vi "Dashboard Main.vi"() -> ()   [LabVIEW 2013]
uses:
  <vilib>/event_ctls.llb/eventvkey.ctl
  <vilib>/Rock Robotics/WPI/Dashboard/WPI_DashboardLogging Global.vi
  <vilib>/Utility/config.llb/Write Key (String).vi
  <vilib>/Utility/config.llb/Write Key (I32).vi
  <vilib>/Utility/config.llb/NI_LVConfig.lvlib
panel:
  out "Image Message":string="Timeout in Camera Communications"
  in  "Rec Mode":enum32{"Stop", "Record", "Playback"}(radio)
  in  "Dashboard Tab":T1(tab)
  in  "Camera Settings":T2={"Frame Rate"=30, "Compression"=30, "Size"=1} {"Frame Rate" scale=1.0..30.0; "Size" items=["640x480", "320x240", "160x120"]}
  out "MotorSliders R":cluster{"MotorSlide1":dbl, "MotorSlide2":dbl} {"MotorSlide2" scale=-1.0..1.0 scale format="%#_2e"; "MotorSlide1" scale=-1.0..1.0 scale format="%#_2e"}
  out "MotorChart R":cluster{"Numeric":dbl, "Numeric":dbl}(graph)
  out "MotorSliders L":T3 {"MotorSlide4 2" scale=0.0..14.0 scale format="%#_2e"; "MotorSlide2" scale=-1.0..1.0 scale format="%#_2e"; "MotorSlide1" scale=-1.0..1.0 scale format="%#_2e"}
  out "MotorChart L":T4(graph)
  out "JS1 Z":dbl(slide) scale=-1.0..1.0 scale format="%#_2e"
  out "Joystick 1":cluster{"X":dbl, "Y":dbl}[](graph)
  out "JS Buttons 1":T5
  out "JS2 Z":dbl(slide) scale=-1.0..1.0 scale format="%#_2e"
  out "Joystick 2":cluster{"X":dbl, "Y":dbl}[](graph)
  out "JS Buttons 2":T5
  out "Mode":T6(ring)=enum."Auto Disabled"
  out "Camera IP":string
  in  "DB Camera Config":bool
  out "fps":dbl format="%#.1g"
  out "Mbps":dbl format="%#.1g"
  out "Mbps 2":bool
  out "LED 1":bool
  out "Time":string
  in  "Slider 1":dbl(slide) scale=0.0..100.0
  in  "Checkbox 2":bool
  in  "Checkbox 1":bool
  in  "Test Slider":dbl(slide) scale=0.0..100.0 scale format="%#_3g"
  in  "On/Off":bool caption="Solenoid"
  in  "Test Name":u16(ring) items=["Select the test to run...", "Example Test", "-------------------------------", "List of tests is built in robot code.", "Replace with your own automated tests."]
  in  "Test Tree":string(tree)
  in  "Motor":cluster{"Value":dbl, "Enable":bool} {"Value" scale=-1.0..1.0 scale format="%#_3g"}
  out "Progress":T7 {"Test Progress" scale=0.0..100.0}
  in  "Rev/Fwd":cluster{"Forward":bool, "Reverse":bool}
  in  "Test Ring":u16(ring) items=["Auto", "Fixed indoor", "Fixed outdoor 1", "Fixed outdoor 2", "Fixed fluorescent 1", "Fixed fluorescent 2", "Hold current"]
  in  "Listbox":i32(listbox)
  out "Tree":string(tree)
  out "Camera Image":T8(plugin-control)
  in  "Enable":bool
  # "Left"
  # "Front"
  # "Right"
  # "Battery"
  # "Customize by placing controls and indicators here and name to\nmatch Dashboard Variables on robot."
  # "This tab is a great place for autonomous settings and validation.\nCustomize by placing controls and indicators here and name to\nmatch Dashboard Variables on robot."
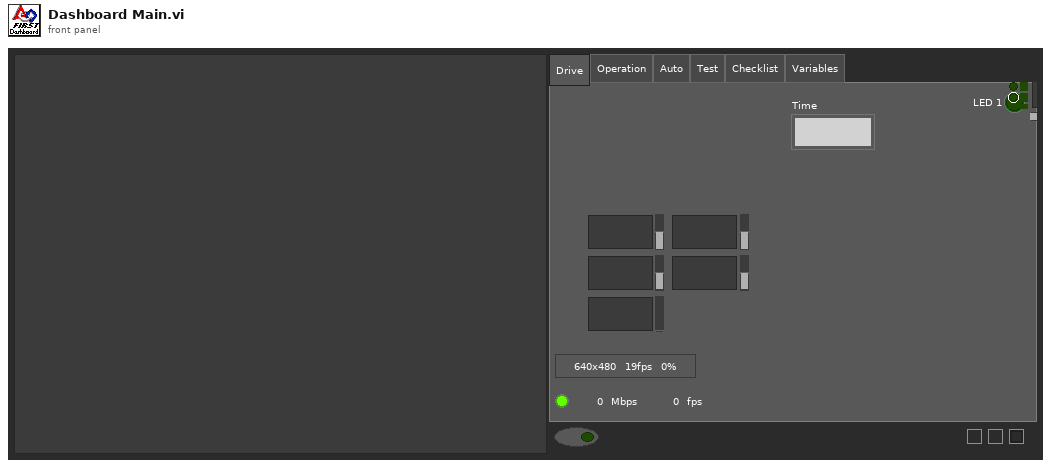
[diagram p1: front panel]
types:
  T1 = enum32{"Drive", "Operation", "Auto", "Test", "Checklist", "Variables"}
  T2 = cluster{"Frame Rate":i32, "Compression":i32, "Size":u16}
  T3 = cluster{"MotorSlide1":dbl, "MotorSlide2":dbl, "MotorSlide4 2":dbl}
  T4 = cluster{"Numeric":dbl, "Numeric":dbl, "Battery":sgl}
  T5 = cluster{bool, bool, bool, bool, bool, bool, bool, bool, bool, bool, bool, bool}
  T6 = enum8{"Tele-Op Disabled", "Tele-Op Enabled", "Auto Disabled", "Auto Enabled", "Test Disabled", "Test Enabled", ""}
  T7 = cluster{"Test Progress":u8, "Test Progress Text":string}
  T8 = typedef "IMAQ Image.ctl" = refnum<image>
  T9 = typedef "Image Type" = u32
  T10 = cluster{"Digital Inputs":bool[], "Digital Outputs":bool[]}
  T11 = cluster{"Competition mode":bool, "Robot Link":bool, "Autonomous":bool, "Enabled":bool, "E-Stop":bool, "Simulated":bool, "TestMode":bool, "Docked Window":bool}
  T12 = cluster{"Boolean Array[0]":bool, "Boolean Array[1]":bool, "Boolean Array[2]":bool, "Boolean Array[3]":bool, "Boolean Array[4]":bool, "Boolean Array[5]":bool, "Boolean Array[6]":bool, "Boolean Array[7]":bool, "Boolean Array[8]":bool, "Boolean Array[9]":bool, "Boolean Array[10]":bool, "Boolean Array[11]":bool}
  T13 = typedef "NI_LVConfig.lvlib/Config Data RefNum.ctl" = refnum<k1>
  T14 = typedef "eventvkey.ctl" = enum16{"ASCII", "Enter", "Return", "Shift", "Ctrl", "Alt", "Cmd", "Opt", "Caps", "NumLock", "Clear", "Break", "Up", "Down", "Left", "Right", "Insert", "Delete", "Home", "End", "PageUp", "PageDown", "Escape", "Help", "Pause", "ScrollLock", "F1", "F2", "F3", "F4", "F5", "F6", "F7", "F8", "F9", "F10", "F11", "F12", "F13", "F14", "F15", "F16", "F17", "F18", "F19", "F20", "F21", "F22", "F23", "F24", "Play", "VolumeUp", "VolumeDown", "Mute", "Two Byte Char"}
  T15 = cluster{"Image Size":bool, "Image Type":bool, "Pixel Value":bool, "ROI Information":bool, "Zoom Factor":bool}
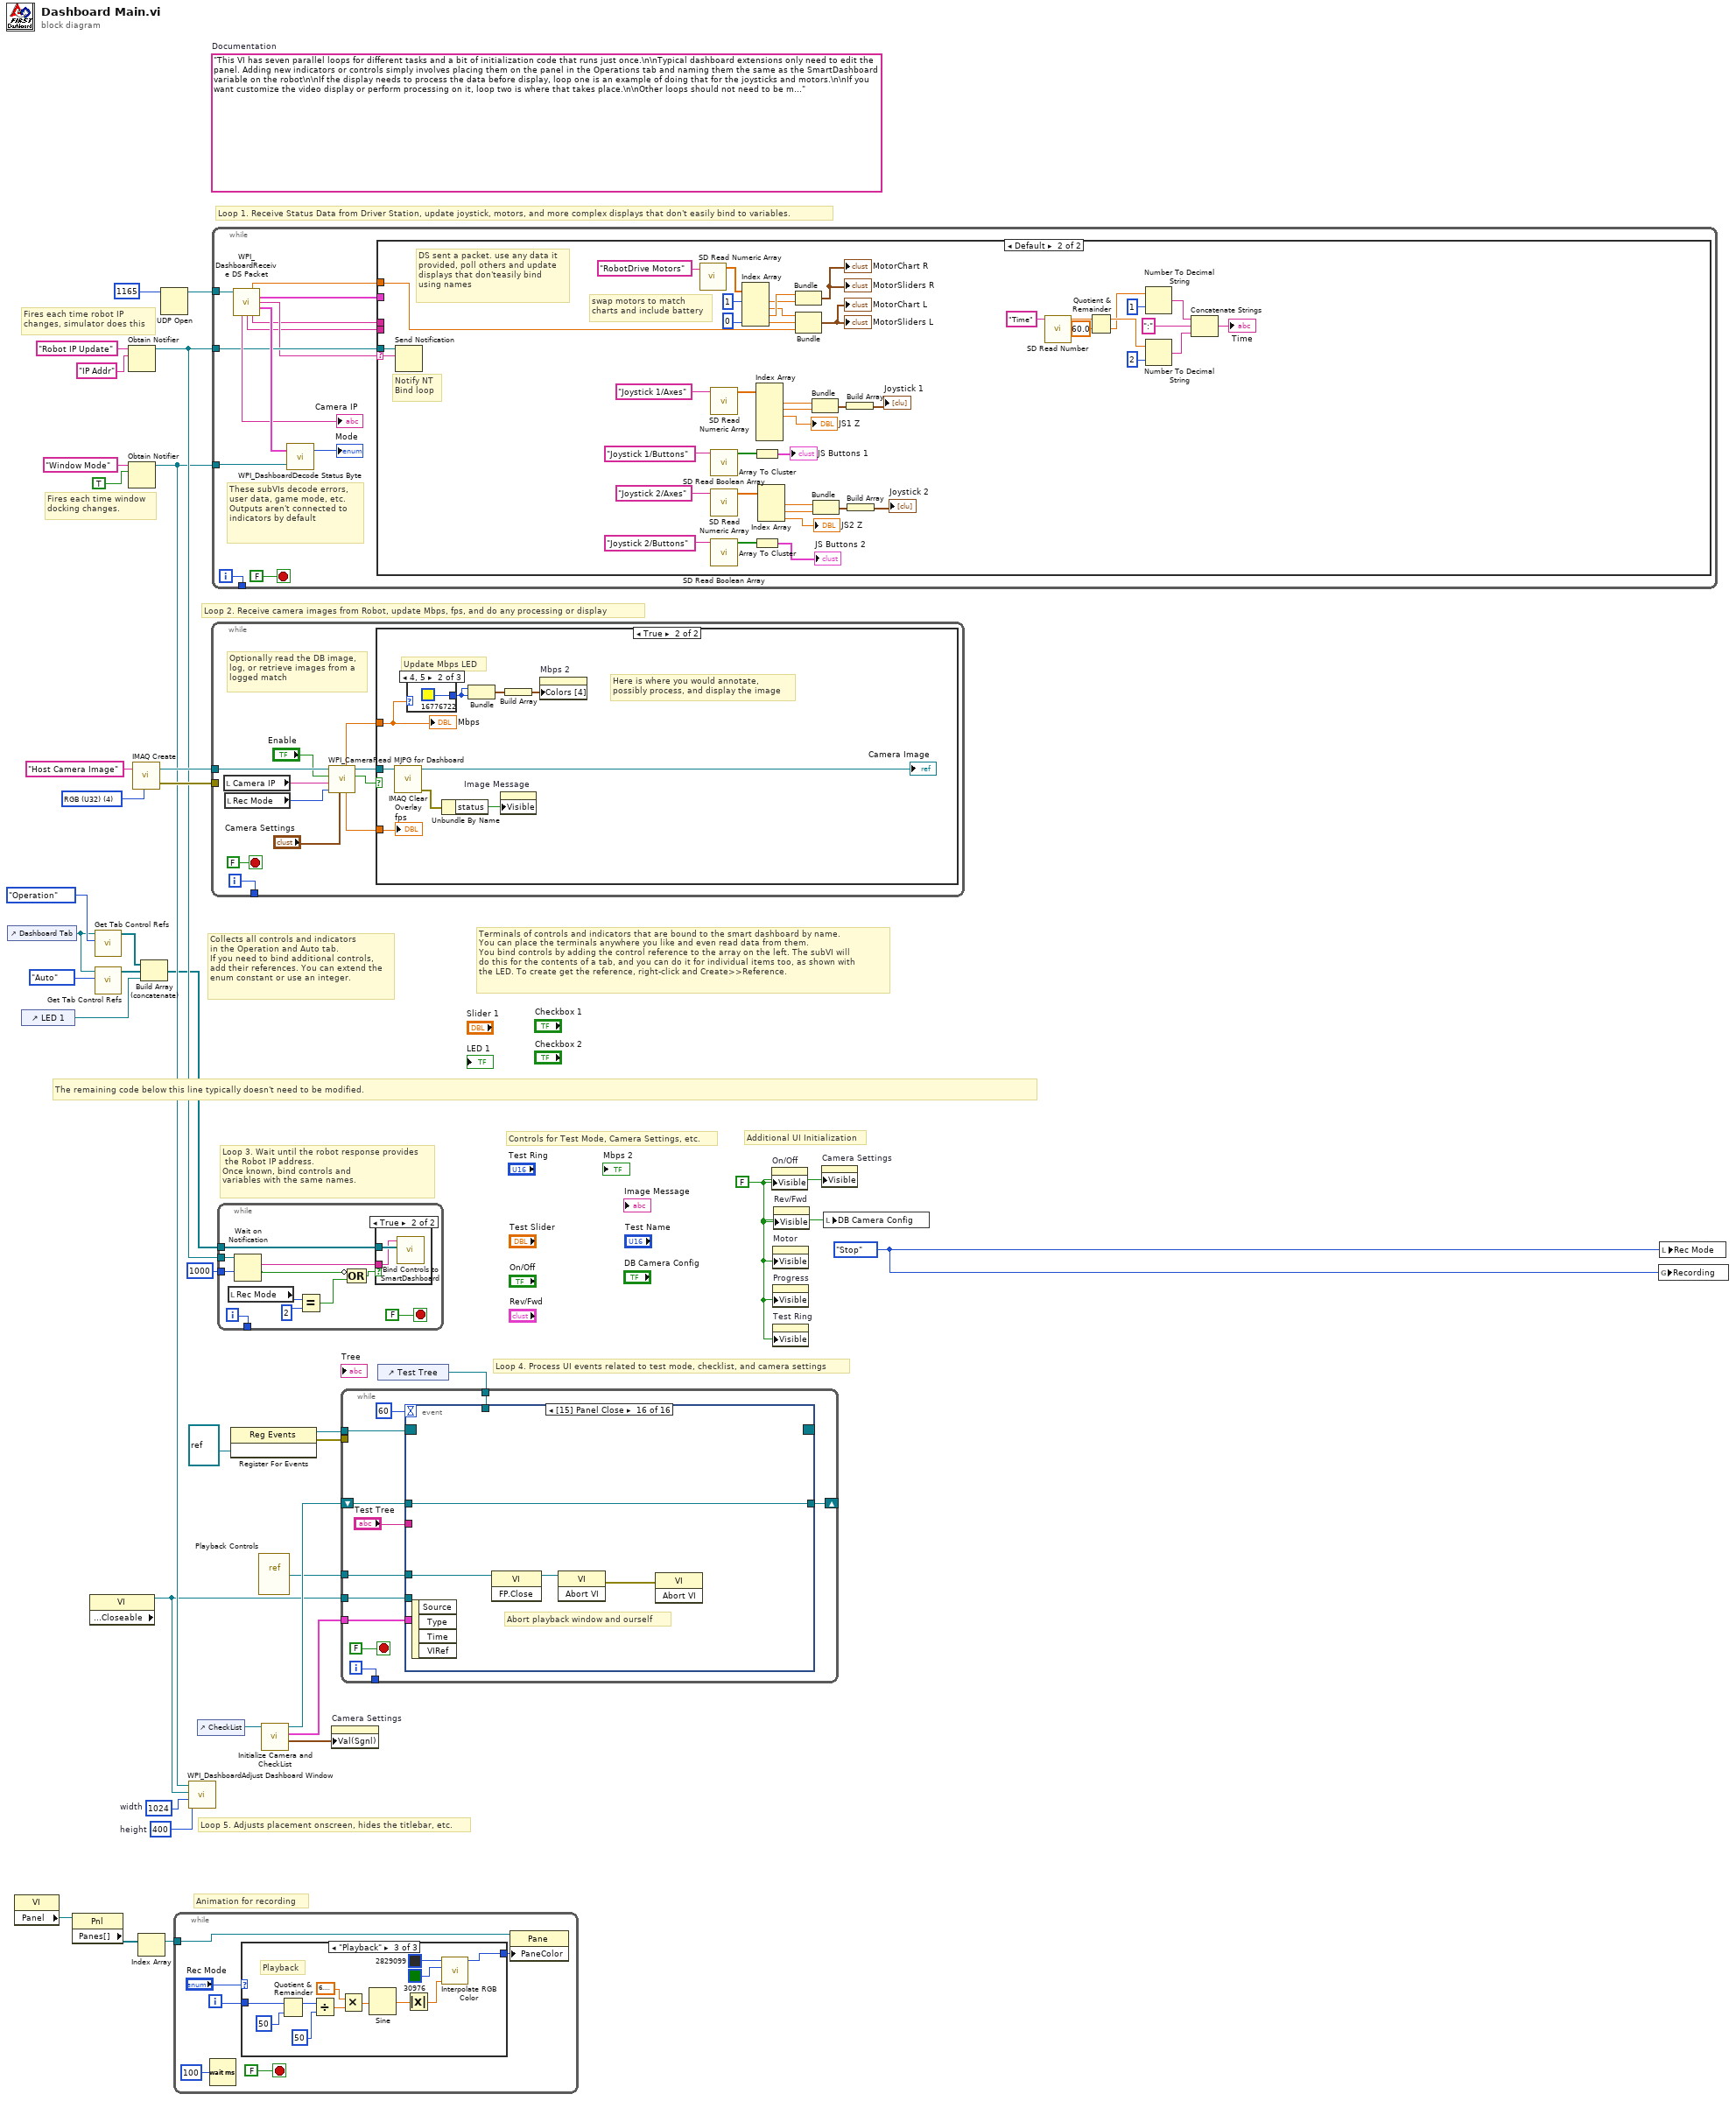
[diagram p0: block diagram]
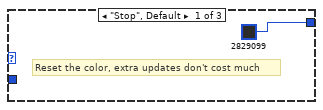
[diagram p2: hidden frame]
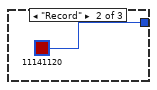
[diagram p3: hidden frame]
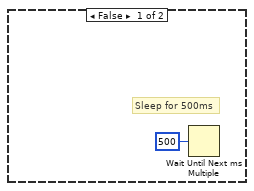
[diagram p5: hidden frame]
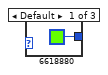
[diagram p6: hidden frame]
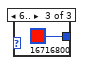
[diagram p7: hidden frame]
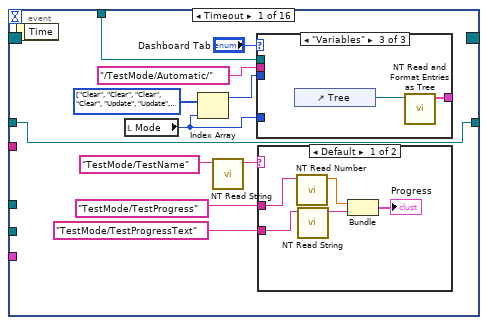
[diagram p8: hidden frame]
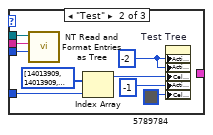
[diagram p10: hidden frame]
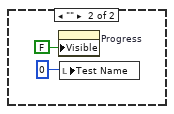
[diagram p11: hidden frame]
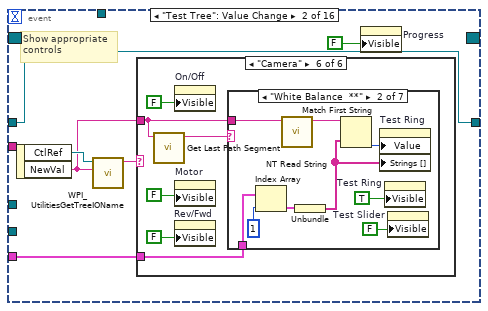
[diagram p12: hidden frame]
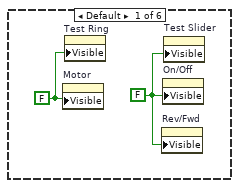
[diagram p13: hidden frame]
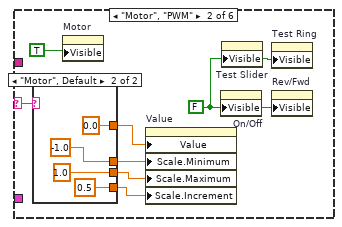
[diagram p14: hidden frame]
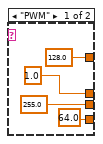
[diagram p15: hidden frame]
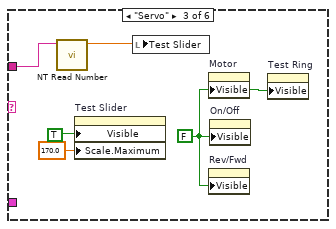
[diagram p16: hidden frame]
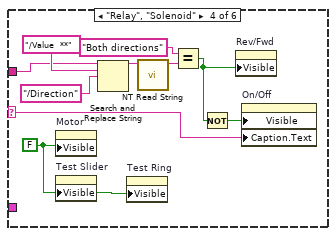
[diagram p17: hidden frame]
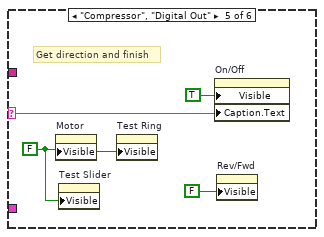
[diagram p18: hidden frame]
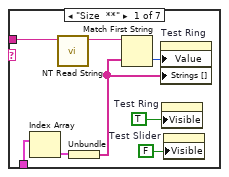
[diagram p19: hidden frame]
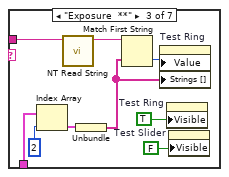
[diagram p20: hidden frame]
diagram:
  w8 = enum32{"Stop", "Record", "Playback"}."Stop" ("Rec Mode")
  w11 = 400  # height
  w12 = 1024  # width
  w25 = FALSE ("Visible")
  (unwired) "This VI has seven parallel loops for different tasks and a bit of initialization code that runs just once.\n\nTypical dashboard extensions only need to edit the panel. Adding new indicators or controls simply involves placing them on the panel in the Operations tab and naming them the same as the SmartDashboard variable on the robot\n\nIf the display needs to process the data before display, loop one is an example of doing that for the joysticks and motors.\n\nIf you want customize the video display or perform processing on it, loop two is where that takes place.\n\nOther loops should not need to be modified. They are pretty standard, and document the task they perform."  # Documentation
  w35 = T9 4 items=["Grayscale (U8)", "Grayscale (I16)", "Grayscale (SGL)", "Complex (CSG)", "RGB (U32)", "HSL (U32)", "RGB (U64)"] ("Image Type")
  # "Controls for Test Mode, Camera Settings, etc."
  # "Additional UI Initialization"
  # "Animation for recording"
  # "Fires each time robot IP\nchanges, simulator does this"
  # "Fires each time window\ndocking changes."
  # "Collects all controls and indicators\nin the Operation and Auto tab.\nIf you need to bind additional controls,\nadd their references. You can extend the\nenum constant or use an integer."
  # "The remaining code below this line typically doesn't need to be modified."
  # "Loop 4. Process UI events related to test mode, checklist, and camera settings"
  # "Terminals of controls and indicators that are bound to the smart dashboard by name.\nYou can place the terminals anywhere you like and even read data from them.\nYou bind controls by adding the control reference to the array on the left. The subVI will\ndo this for the contents of a tab, and you can do it for individual items too, as shown with\nthe LED. To create get the reference, right-click and Create>>Reference."
  # "Loop 3. Wait until the robot response provides\n the Robot IP address.\nOnce known, bind controls and\nvariables with the same names."
  # "Loop 5. Adjusts placement onscreen, hides the titlebar, etc."
  # "Loop 1. Receive Status Data from Driver Station, update joystick, motors, and more complex displays that don't easily bind to variables."
  # "Loop 2. Receive camera images from Robot, update Mbps, fps, and do any processing or display"
  n1 = control-ref of="Dashboard Tab"() -> (w6:refnum<vi>)
  n2 = property class="VI"() -> ("Panel"=w19:refnum<vi>)  [unwired: 2 in, 2 out]
  n3 = control-ref of="LED 1"() -> (w1:refnum<vi>)
  n4 = property class="Pnl"(reference=w19) -> ("Panes[]"=w20:refnum<vi>[])  [unwired: 1 in, 2 out]
  n5 = property class="VI" props=["Front Panel.Closeable"]() -> (reference out=w7:refnum<vi>)  [unwired: 2 in, 2 out]
  n6 = call <vilib>:"Get Tab Control Refs.vi"("Page Index"=T1."Operation" ("Dashboard Tab"), "TabControl in"=w6) -> ("ControlsOnPage"=w4:refnum<vi>[])  [unwired: 9 in]
  n7 = call <vilib>:"Get Tab Control Refs.vi"("Page Index"=T1."Auto" ("Dashboard Tab"), "TabControl in"=w6) -> ("ControlsOnPage"=w5:refnum<vi>[])  [unwired: 9 in]
  n8 = Obtain Notifier(name (unnamed)="Robot IP Update", notification data type="IP Addr" ("name (unnamed)")) -> (notifier out=w29:refnum<notifier>)  [unwired: 2 in, 2 out]
  n9 = Obtain Notifier(name (unnamed)="Window Mode", notification data type=TRUE) -> (notifier out=w10:refnum<notifier>)  [unwired: 2 in, 2 out]
  n10 = call "IMAQ Create"("Image Name"="Host Camera Image", "Image Type"=w35) -> ("New Image"=w33:T8, "error out"=w32:errorcluster)  [unwired: 2 in, 1 out]
  n11 = Index Array(array=w20) -> (element=w18:refnum<vi>)  [unwired: 1 in]
  n12 = Build Array (concatenate)(w4, w5, w1) -> (w3:refnum<vi>[])
  n13 = UDP Open(11:u16 1165 ("port")) -> (port=w36:refnum<k16>)  [unwired: 2 in, 4 out]
  n14 = while {
    tunnel: w18 -> [w39]
    i -> [w42]
    stop <- FALSE stop-if-true
    n15 = Wait (ms)(milliseconds to wait=u32 100) -> ()  [unwired: 1 out]
    n16 = case shown="\"Playback\"" "Rec Mode" {
      tunnel: w42 -> [_ _ w57]
      tunnel: [u32 2829099 ("Base Color") u32 11141120 ("Target Color") w46] -> w38
      frame "Stop", Default {
        # "Reset the color, extra updates don't cost much"
      }
      frame "Record" {
      }
      frame "Playback" {
        # "Playback"
        n17 = Quotient & Remainder(x=w57, y=u32 50 ("milliseconds to wait")) -> (x-y*floor(x/y)=w53:u32)  [unwired: 1 out]
        n18 = Divide(x=w53, y=u32 50 ("milliseconds to wait")) -> (x/y=w50:dbl)
        n19 = Multiply(x=6.283185307179586, y=w50) -> (x*y=w55:dbl)
        n20 = Sine(x=w55) -> (sin(x)=w54:dbl)
        n21 = Absolute Value(x=w54) -> (abs(x)=w47:dbl)
        n22 = call "Interpolate RGB Color.vi"("Proportion"=w47, "Target Color"=u32 30976, "Base Color"=u32 2829099) -> ("Result Color"=w46:u32)  [unwired: 8 in]
      }
    }
    n23 = property class="Pane"(reference=w39, "PaneColor"=w38) -> ()  [unwired: 1 in, 2 out]
  }
  n24 = call <vilib>:"WPI_DashboardAdjust Dashboard Window.vi"("height"=w11, "width"=w12, "reference in"=w7, "Notifier in"=w10) -> ()  [unwired: 8 in]
  n25 = control-ref of="CheckList"() -> (w9:refnum<vi>)
  n26 = while {
    tunnel: w33 -> [w66]
    tunnel: w32 -> [_]
    tunnel: [w67] -> _
    i -> [w67]
    stop <- FALSE stop-if-true
    # "Optionally read the DB image,\nlog, or retrieve images from a\nlogged match"
    n27 = local read "Camera IP"() -> (w59:string)
    n28 = local read "Rec Mode"() -> (w58:enum32{"Stop", "Record", "Playback"})
    n29 = call <vilib>:"WPI_CameraRead MJPG for Dashboard.vi"("Camera Settings"="Camera Settings", "Rec Mode"=w58, "Camera IP"=w59, "Enable"="Enable", "Refnum in"=w66) -> ("Active"=w63:bool, "Refnum out"=w65:T8, "FPS"=w62:dbl, "Bandwidth (Mbps)"=w61:dbl)  [unwired: 3 in]
    n30 = case shown="True" w63 {
      tunnel: w65 -> [_ w73]
      tunnel: w61 -> [_ w72]
      tunnel: w62 -> [_ w70]
      frame False {
        # "Sleep for 500ms"
        n31 = Wait Until Next ms Multiple(millisecond multiple=u32 500) -> ()  [unwired: 1 out]
      }
      frame True {
        # "Here is where you would annotate,\npossibly process, and display the image"
        # "Update Mbps LED"
        n32 = call "IMAQ Clear Overlay"("Image"=w73) -> ("error out"=w77:errorcluster, "Image Out"=→"Camera Image":T8)  [unwired: 2 in, 7 out]
        n33 = case shown="4, 5" w72 {
          tunnel: [u32 6618880 ("Color Box") u32 16776722 ("Color Box") u32 16716800 ("Color Box")] -> w74
          frame Default {
          }
          frame 4, 5 {
          }
          frame 6.. {
          }
        }
        n34 = Unbundle By Name(w77) -> ("status"=w78:bool)
        n35 = Bundle("Color Box"=w74, "Color Box"=w74) -> (w76:cluster{"Color Box":u32, "Color Box":u32})  [unwired: 1 out]
        n36 = property on="Image Message" class="Str"("Visible"=w78) -> ()  [unwired: 2 in, 2 out]
        n37 = Build Array(w76) -> (w75:cluster{"Color Box":u32, "Color Box":u32}[])
        n38 = property on="Mbps 2" class="Bool (strict)"("Colors [4]"=w75) -> ()  [unwired: 2 in, 2 out]
        "Mbps" <- w72
        "fps" <- w70
      }
    }
  }
  n39 = while {
    tunnel: w36 -> [w92]
    tunnel: w29 -> [w87]
    tunnel: w10 -> [w91]
    tunnel: [w88] -> _
    i -> [w88]
    stop <- FALSE stop-if-true
    # "These subVIs decode errors, user data, game mode, etc.\nOutputs aren't connected to indicators by default"
    n40 = call <vilib>:"WPI_DashboardReceive DS Packet.vi"("Recv Socket"=w92) -> ("Battery"=w82:sgl, "Driver Station"=w83:T10, "Robot IP Address"=w86:string, "Status"=w93:T11, "Camera IP Address"=→"Camera IP":string, "Low Priority User Data"=w85:string, "High Priority User Data"=w84:string)  [unwired: 1 in, 7 out]
    n41 = call <vilib>:"WPI_DashboardDecode Status Byte.vi"("Window Mode Notifier"=w91, "Status"=w93) -> ("Mode"=→"Mode":T6)  [unwired: 1 out]
    n42 = case shown="Default" w86 {
      selector: w86 -> [_ w116]
      tunnel: w87 -> [_ w117]
      tunnel: w85 -> [_ _]
      tunnel: w84 -> [_ _]
      tunnel: w83 -> [_ _]
      tunnel: w82 -> [_ w115]
      frame "0.0.0.0" {
        # "DS not sending packets, or no robot exists yet.\nDon't poll the variables"
      }
      frame Default {
        # "Notify NT\nBind loop"
        # "DS sent a packet. use any data it\nprovided, poll others and update\ndisplays that don'teasily bind\nusing names"
        # "swap motors to match\ncharts and include battery"
        n43 = Send Notification(notification=w116, notifier=w117) -> ()  [unwired: 1 in, 2 out]
        n44 = call <vilib>:"SD Read Numeric Array.vi"("Name"="RobotDrive Motors") -> ("Numeric Array"=w114:dbl[])  [unwired: 8 in, 2 out]
        n45 = call <vilib>:"SD Read Numeric Array.vi"("Name"="Joystick 1/Axes") -> ("Numeric Array"=w133:dbl[])  [unwired: 8 in, 2 out]
        n46 = call <vilib>:"SD Read Boolean Array.vi"("Name"="Joystick 1/Buttons") -> ("Boolean Array"=w135:bool[])  [unwired: 8 in, 2 out]
        n47 = call <vilib>:"SD Read Numeric Array.vi"("Name"="Joystick 2/Axes") -> ("Numeric Array"=w127:dbl[])  [unwired: 8 in, 2 out]
        n48 = call <vilib>:"SD Read Boolean Array.vi"("Name"="Joystick 2/Buttons") -> ("Boolean Array"=w126:bool[])  [unwired: 8 in, 2 out]
        n49 = Index Array(array=w114, index #1=1, index #4=0) -> (element #1=w110:dbl, element #2=w109:dbl, element #3=w111:dbl, element #4=w106:dbl)  [unwired: 2 in]
        n50 = Array To Cluster(array=w135) -> (cluster=→"JS Buttons 1":T12)
        n51 = Array To Cluster(array=w126) -> (cluster=→"JS Buttons 2":T12)
        n52 = Index Array(array=w133) -> (element #1=w130:dbl, element #2=w131:dbl, element #3=→"JS1 Z":dbl)  [unwired: 6 in, 3 out]
        n53 = Index Array(array=w127) -> (element #1=w122:dbl, element #2=w121:dbl, element #3=→"JS2 Z":dbl)  [unwired: 3 in]
        n54 = Bundle("Numeric"=w111, "Numeric"=w110) -> (→"MotorChart R" →"MotorSliders R":cluster{"Numeric":dbl, "Numeric":dbl})  [unwired: 1 in]
        n55 = Bundle("Numeric"=w109, "Numeric"=w106, "Battery"=w115) -> (→"MotorChart L" →"MotorSliders L":T4)  [unwired: 1 in]
        n56 = Bundle("Numeric"=w130, "Numeric"=w131) -> (w129:cluster{"Numeric":dbl, "Numeric":dbl})  [unwired: 1 in]
        n57 = Bundle("Numeric"=w122, "Numeric"=w121) -> (w123:cluster{"Numeric":dbl, "Numeric":dbl})  [unwired: 1 in]
        n58 = Build Array(w129) -> (→"Joystick 1":cluster{"Numeric":dbl, "Numeric":dbl}[])
        n59 = Build Array(w123) -> (→"Joystick 2":cluster{"Numeric":dbl, "Numeric":dbl}[])
        n60 = call <vilib>:"SD Read Number.vi"("Name"="Time") -> ("Numeric"=w104:dbl)  [unwired: 8 in, 2 out]
        n61 = Quotient & Remainder(x=w104, y=60.0) -> (x-y*floor(x/y)=w99:dbl, floor(x/y)=w96:dbl)
        n62 = Number To Decimal String(number=w96, width (-)=i16 1) -> (decimal integer string=w102:string)
        n63 = Number To Decimal String(number=w99, width (-)=i16 2) -> (decimal integer string=w101:string)
        n64 = Concatenate Strings(w102, ":", w101) -> (→"Time":string)
      }
    }
  }
  n65 = while {
    tunnel: w3 -> [w149]
    tunnel: w29 -> [w147]
    tunnel: [w145] -> _
    tunnel: u32 1000 ("milliseconds to wait") -> [w144]
    i -> [w145]
    stop <- FALSE stop-if-true
    n66 = local read "Rec Mode"() -> (w140:enum32{"Stop", "Record", "Playback"})
    n67 = Wait on Notification(notifier=w147, timeout in ms (-1)=w144) -> (notification=w146:string, timed out?=w142:bool)  [unwired: 2 in, 2 out]
    n68 = Equal?(x=w140, y=u16 2 ("Rec Mode")) -> (x = y?=w141:bool)
    n69 = Compound Arithmetic op=OR(invert w142, w141) -> (w143:bool)
    n70 = case shown="True" w143 {
      tunnel: w149 -> [_ w151]
      tunnel: w146 -> [_ w150]
      frame False {
      }
      frame True {
        n71 = call <vilib>:"Bind Controls to SmartDashboard.vi"("Bound Control Refs"=w151, "Server IP Address"=w150) -> ()  [unwired: 10 in]
      }
    }
  }
  n72 = register-events(refnum<vi> refnum) -> (reference out=w16:refnum<event-registration>, error out=w15:errorcluster)  [unwired: 2 in]
  n73 = vi-ref "Playback Controls.vi"() -> (w17:refnum<vi>)
  n74 = call "Initialize Camera and CheckList.vi"("ListBox in"=w9) -> ("Cluster"=w23:cluster{"value":i32, "value":i32, "index":i32}, "Array"=w24:cluster{string[]}[], "File Refnum"=w22:T13)  [unwired: 8 in]
  n75 = property on="Camera Settings" class="Clust (strict)"("Val(Sgnl)"=w23) -> ()  [unwired: 2 in, 2 out]
  n76 = control-ref of="Test Tree"() -> (w21:refnum<vi>)
  n77 = while {
    tunnel: w24 -> [w159]
    shift-right: [w158] -> _
    shift-left: w22 -> [w157]
    tunnel: [w156] -> _
    tunnel: w21 -> [w155]
    tunnel: w17 -> [w154]
    tunnel: w16 -> [w153]
    tunnel: w15 -> [_]
    tunnel: w7 -> [w152]
    i -> [w156]
    stop <- FALSE stop-if-true
    n78 = event shown="[15] Panel Close" {
      selector: w153 -> [_ _ _ _ _ _ _ _ _ _ _ _ _ _ _ _]
      dyn-events: [_ _ _ _ _ _ _ _ _ _ _ _ _ w397 _ _] -> _
      timeout: u32 60 ("milliseconds to wait") -> [_ _ _ _ _ _ _ _ _ _ _ _ _ _ _ _]
      tunnel: w155 -> [w169 _ _ _ _ _ _ _ _ _ _ _ _ _ _ _]
      tunnel: "Test Tree" -> [_ _ _ _ _ _ _ _ w366 w374 w376 w380 w388 _ _ _]
      tunnel: w159 -> [_ w193 _ _ _ _ w330 w360 _ _ _ _ _ _ _ _]
      tunnel: [w163 w192 w291 w296 w304 w316 w329 w353 w365 w372 w375 w379 w387 w399 w413 w414] -> w158
      tunnel: w157 -> [w163 w192 w291 w296 w304 w316 w328 w353 w365 w372 w375 w379 w387 w399 w413 w414]
      tunnel: w154 -> [_ _ _ _ _ _ _ _ _ _ _ _ _ w400 _ w417]
      tunnel: w152 -> [_ _ _ _ _ _ _ _ _ _ _ _ _ w395 _ _]
      event Timeout {
        w168 = enum16{"Update", "Clear"}[] [enum."Clear", enum."Clear", enum."Clear", enum."Clear", enum."Update", enum."Update", enum."Clear"] items=["Update", "Clear"]
        n79 = event-data() -> ()  [unwired: 1 in, 1 out]
        n80 = local read "Mode"() -> (w166:T6)
        n81 = Index Array(array=w168, index=w166) -> (element=w167:enum16{"Update", "Clear"})
        n82 = call <vilib>:"NT Read String.vi"("Name"="TestMode/TestName") -> ("String"=w172:string)  [unwired: 9 in, 1 out]
        n83 = case shown="\"Variables\"" "Dashboard Tab" {
          tunnel: w169 -> [_ w182 _]
          tunnel: "/TestMode/Automatic/" ("Name Pattern") -> [_ w181 _]
          tunnel: w167 -> [_ w180 _]
          tunnel: w166 -> [_ w178 _]
          tunnel: [_ _ w184] -> _
          frame "Operation", Default {
          }
          frame "Test" {
            w177 = -2 ("Active Item:Row Number")
            n84 = call <vilib>:"NT Read and Format Entries as Tree.vi"("Operation"=w180, "Name Pattern"=w181, "Tree Refnum"=w182) -> ()  [unwired: 7 in, 2 out]
            n85 = Index Array(array=u32[] [14013909, 14013909, 14013909, 14013909, 14013909, 16777215, 14013909], index=w178) -> (element=w176:u32)
            n86 = property on="Test Tree" class="Tree (strict)"("Active Item Row Number"=w177, "ActiveColNum"=w177, "CellBG"=w176, "Active Item Row Number"=-1 ("Active Item:Row Number"), "CellBG"=u32 5789784 ("Color Box")) -> ()  [unwired: 2 in, 2 out]
          }
          frame "Variables" {
            n87 = control-ref of="Tree"() -> (w183:refnum<vi>)
            n88 = call <vilib>:"NT Read and Format Entries as Tree.vi"("Tree Refnum"=w183) -> ("Formatted Strings"=w184:cluster{"Name":string, "Value":string}[])  [unwired: 9 in, 1 out]
          }
        }
        n89 = case shown="Default" w172 {
          tunnel: "TestMode/TestProgress" ("Name") -> [w186 _]
          tunnel: "TestMode/TestProgressText" ("Name") -> [w185 _]
          frame Default {
            n90 = call <vilib>:"NT Read Number.vi"("Name"=w186) -> ("Numeric"=w187:dbl)  [unwired: 9 in, 1 out]
            n91 = call <vilib>:"NT Read String.vi"("Name"=w185) -> ("String"=w188:string)  [unwired: 9 in, 1 out]
            n92 = Bundle("Numeric"=w187, "String"=w188) -> (→"Progress":cluster{"Numeric":dbl, "String":string})  [unwired: 1 in]
          }
          frame "" {
            n93 = property on="Progress" class="Clust (strict)"("Visible"=FALSE) -> ()  [unwired: 2 in, 2 out]
            n94 = local write "Test Name"(u16 0) -> ()
          }
        }
      }
      event "Test Tree": Value Change {
        # "Show appropriate\ncontrols"
        n95 = event-data() -> ("CtlRef"=w196:refnum<vi>, "NewVal"=w194:string)  [unwired: 1 in]
        n96 = call <vilib>:"WPI_UtilitiesGetTreeIOName.vi"("NewVal"=w194, "TreeControl in"=w196) -> ("I/O Name"=w197:string)  [unwired: 9 in]
        n97 = case shown="\"Camera\"" w197 {
          selector: w197 -> [_ w204 _ w222 w231 _]
          tunnel: w194 -> [_ _ w219 w221 _ w238]
          tunnel: w193 -> [_ _ _ _ _ w237]
          frame Default {
            w199 = FALSE ("Visible")
            w198 = FALSE ("Visible")
            n98 = property on="Motor" class="Clust (strict)"("Visible"=w198) -> ()  [unwired: 2 in, 2 out]
            n99 = property on="Test Ring" class="Ring (strict)"("Visible"=w198) -> ()  [unwired: 2 in, 2 out]
            n100 = property on="Rev/Fwd" class="Clust (strict)"("Visible"=w199) -> ()  [unwired: 2 in, 2 out]
            n101 = property on="On/Off" class="Bool (strict)"("Visible"=w199) -> ()  [unwired: 2 in, 2 out]
            n102 = property on="Test Slider" class="Slide (strict)"("Visible"=w199) -> ()  [unwired: 2 in, 2 out]
          }
          frame "Motor", "PWM" {
            w205 = FALSE ("Visible")
            n103 = case shown="\"Motor\", Default" w204 {
              tunnel: [1.0 ("Value") -1.0 ("Value")] -> w203
              tunnel: [255.0 ("Value") 1.0 ("Value")] -> w202
              tunnel: [128.0 ("Value") 0.0 ("Value")] -> w201
              tunnel: [64.0 ("Value") 0.5 ("Value")] -> w200
              frame "PWM" {
              }
              frame "Motor", Default {
              }
            }
            n104 = property on="Motor" class="Clust (strict)"("Visible"=TRUE) -> ()  [unwired: 2 in, 2 out]
            n105 = property on="Value" class="Slide (strict)"("Value"=w201, "Scale.Minimum"=w203, "Scale.Maximum"=w202, "Scale.Increment"=w200) -> ()  [unwired: 2 in, 2 out]
            n106 = property on="On/Off" class="Bool (strict)"("Visible"=w205) -> ()  [unwired: 2 in, 2 out]
            n107 = property on="Test Slider" class="Slide (strict)"("Visible"=w205) -> ()  [unwired: 2 in, 2 out]
            n108 = property on="Test Ring" class="Ring (strict)"("Visible"=w205) -> ()  [unwired: 2 in, 2 out]
            n109 = property on="Rev/Fwd" class="Clust (strict)"("Visible"=w205) -> ()  [unwired: 2 in, 2 out]
          }
          frame "Servo" {
            w217 = FALSE ("Visible")
            n110 = call <vilib>:"NT Read Number.vi"("Name"=w219) -> ("Numeric"=w218:dbl)  [unwired: 9 in, 1 out]
            n111 = property on="Test Slider" class="Slide (strict)"("Visible"=TRUE, "Scale.Maximum"=170.0 ("Scale.Range:Maximum")) -> ()  [unwired: 2 in, 2 out]
            n112 = local write "Test Slider"(w218) -> ()
            n113 = property on="Motor" class="Clust (strict)"("Visible"=w217) -> ()  [unwired: 2 in, 2 out]
            n114 = property on="Rev/Fwd" class="Clust (strict)"("Visible"=w217) -> ()  [unwired: 2 in, 2 out]
            n115 = property on="On/Off" class="Bool (strict)"("Visible"=w217) -> ()  [unwired: 2 in, 2 out]
            n116 = property on="Test Ring" class="Ring (strict)"("Visible"=w217) -> ()  [unwired: 2 in, 2 out]
          }
          frame "Relay", "Solenoid" {
            w220 = FALSE ("Visible")
            n117 = property on="Motor" class="Clust (strict)"("Visible"=w220) -> ()  [unwired: 2 in, 2 out]
            n118 = property on="Test Slider" class="Slide (strict)"("Visible"=w220) -> ()  [unwired: 2 in, 2 out]
            n119 = Search and Replace String(input string=w221, search string="/Value  **", replace string="/Direction") -> (result string=w227:string)  [unwired: 5 in, 3 out]
            n120 = property on="Test Ring" class="Ring (strict)"("Visible"=w220) -> ()  [unwired: 2 in, 2 out]
            n121 = call <vilib>:"NT Read String.vi"("Name"=w227) -> ("String"=w225:string)  [unwired: 9 in, 1 out]
            n122 = Equal?(x="Both directions", y=w225) -> (x = y?=w223:bool)
            n123 = Not(x=w223) -> (.not. x?=w224:bool)
            n124 = property on="Rev/Fwd" class="Clust (strict)"("Visible"=w223) -> ()  [unwired: 2 in, 2 out]
            n125 = property on="On/Off" class="Bool (strict)"("Visible"=w224, "Caption.Text"=w222) -> ()  [unwired: 2 in, 2 out]
          }
          frame "Compressor", "Digital Out" {
            w230 = FALSE ("Visible")
            # "Get direction and finish"
            n126 = property on="Motor" class="Clust (strict)"("Visible"=w230) -> ()  [unwired: 2 in, 2 out]
            n127 = property on="Test Slider" class="Slide (strict)"("Visible"=w230) -> ()  [unwired: 2 in, 2 out]
            n128 = property on="Test Ring" class="Ring (strict)"("Visible"=w230) -> ()  [unwired: 2 in, 2 out]
            n129 = property on="On/Off" class="Bool (strict)"("Visible"=TRUE, "Caption.Text"=w231) -> ()  [unwired: 2 in, 2 out]
            n130 = property on="Rev/Fwd" class="Clust (strict)"("Visible"=FALSE) -> ()  [unwired: 2 in, 2 out]
          }
          frame "Camera" {
            n131 = call <vilib>:"Get Last Path Segment.vi"("String in"=w238) -> ("String out"=w239:string)  [unwired: 10 in]
            n132 = property on="On/Off" class="Bool (strict)"("Visible"=FALSE) -> ()  [unwired: 2 in, 2 out]
            n133 = property on="Motor" class="Clust (strict)"("Visible"=FALSE) -> ()  [unwired: 2 in, 2 out]
            n134 = property on="Rev/Fwd" class="Clust (strict)"("Visible"=FALSE) -> ()  [unwired: 2 in, 2 out]
            n135 = case shown="\"White Balance  **\"" w239 {
              tunnel: w238 -> [w245 w254 w263 w272 w281 _ w287]
              tunnel: w237 -> [w243 w251 w260 w269 w278 _ _]
              frame "Size  **" {
                n136 = Index Array(array=w243) -> (element=w242:cluster{string[]})  [unwired: 1 in]
                n137 = call <vilib>:"NT Read String.vi"("Name"=w245) -> ("String"=w244:string)  [unwired: 9 in, 1 out]
                n138 = Unbundle(w242) -> (w240:string[])
                n139 = Match First String(2:w240, 3:w244) -> (0:w241:i32)  [unwired: 1 out]
                n140 = property on="Test Ring" class="Ring (strict)"("Value"=w241, "Strings []"=w240) -> ()  [unwired: 2 in, 2 out]
                n141 = property on="Test Ring" class="Ring (strict)"("Visible"=TRUE) -> ()  [unwired: 2 in, 2 out]
                n142 = property on="Test Slider" class="Slide (strict)"("Visible"=FALSE) -> ()  [unwired: 2 in, 2 out]
              }
              frame "White Balance  **" {
                n143 = Index Array(array=w251, index=1) -> (element=w252:cluster{string[]})
                n144 = call <vilib>:"NT Read String.vi"("Name"=w254) -> ("String"=w253:string)  [unwired: 9 in, 1 out]
                n145 = Unbundle(w252) -> (w249:string[])
                n146 = Match First String(2:w249, 3:w253) -> (0:w248:i32)  [unwired: 1 out]
                n147 = property on="Test Ring" class="Ring (strict)"("Value"=w248, "Strings []"=w249) -> ()  [unwired: 2 in, 2 out]
                n148 = property on="Test Ring" class="Ring (strict)"("Visible"=TRUE) -> ()  [unwired: 2 in, 2 out]
                n149 = property on="Test Slider" class="Slide (strict)"("Visible"=FALSE) -> ()  [unwired: 2 in, 2 out]
              }
              frame "Exposure  **" {
                n150 = Index Array(array=w260, index=2) -> (element=w261:cluster{string[]})
                n151 = call <vilib>:"NT Read String.vi"("Name"=w263) -> ("String"=w262:string)  [unwired: 9 in, 1 out]
                n152 = Unbundle(w261) -> (w257:string[])
                n153 = Match First String(2:w257, 3:w262) -> (0:w258:i32)  [unwired: 1 out]
                n154 = property on="Test Ring" class="Ring (strict)"("Value"=w258, "Strings []"=w257) -> ()  [unwired: 2 in, 2 out]
                n155 = property on="Test Ring" class="Ring (strict)"("Visible"=TRUE) -> ()  [unwired: 2 in, 2 out]
                n156 = property on="Test Slider" class="Slide (strict)"("Visible"=FALSE) -> ()  [unwired: 2 in, 2 out]
              }
              frame "Exposure Priority  **" {
                n157 = Index Array(array=w269, index=3) -> (element=w270:cluster{string[]})
                n158 = call <vilib>:"NT Read String.vi"("Name"=w272) -> ("String"=w271:string)  [unwired: 9 in, 1 out]
                n159 = Unbundle(w270) -> (w266:string[])
                n160 = Match First String(2:w266, 3:w271) -> (0:w267:i32)  [unwired: 1 out]
                n161 = property on="Test Ring" class="Ring (strict)"("Value"=w267, "Strings []"=w266) -> ()  [unwired: 2 in, 2 out]
                n162 = property on="Test Ring" class="Ring (strict)"("Visible"=TRUE) -> ()  [unwired: 2 in, 2 out]
                n163 = property on="Test Slider" class="Slide (strict)"("Visible"=FALSE) -> ()  [unwired: 2 in, 2 out]
              }
              frame "Color Enable  **" {
                n164 = Index Array(array=w278, index=4) -> (element=w279:cluster{string[]})
                n165 = call <vilib>:"NT Read String.vi"("Name"=w281) -> ("String"=w280:string)  [unwired: 9 in, 1 out]
                n166 = Unbundle(w279) -> (w275:string[])
                n167 = Match First String(2:w275, 3:w280) -> (0:w276:i32)  [unwired: 1 out]
                n168 = property on="Test Ring" class="Ring (strict)"("Value"=w276, "Strings []"=w275) -> ()  [unwired: 2 in, 2 out]
                n169 = property on="Test Ring" class="Ring (strict)"("Visible"=TRUE) -> ()  [unwired: 2 in, 2 out]
                n170 = property on="Test Slider" class="Slide (strict)"("Visible"=FALSE) -> ()  [unwired: 2 in, 2 out]
              }
              frame Default {
                n171 = property on="Test Ring" class="Ring (strict)"("Visible"=FALSE) -> ()  [unwired: 2 in, 2 out]
                n172 = property on="Test Slider" class="Slide (strict)"("Visible"=FALSE) -> ()  [unwired: 2 in, 2 out]
              }
              frame "Brightness  **", "Color Level  **", "Compression  **", "FPS  **", "Sharpness  **" {
                n173 = call <vilib>:"NT Read Number.vi"("Name"=w287) -> ("Numeric"=w286:dbl)  [unwired: 9 in, 1 out]
                n174 = local write "Test Slider"(w286) -> ()
                n175 = property on="Test Slider" class="Slide (strict)"("Visible"=TRUE, "Scale.Maximum"=100.0 ("Scale.Range:Maximum")) -> ()  [unwired: 2 in, 2 out]
                n176 = property on="Test Ring" class="Ring (strict)"("Visible"=FALSE) -> ()  [unwired: 2 in, 2 out]
              }
            }
          }
        }
        n177 = property on="Progress" class="Clust (strict)"("Visible"=FALSE) -> ()  [unwired: 2 in, 2 out]
      }
      event "Test Name": Mouse Enter {
        # "Populate the ring with the list of tests"
        n178 = event-data() -> ()  [unwired: 1 in, 1 out]
        n179 = call <vilib>:"NT Read String Array.vi"("Name"="TestMode/TestList") -> ("String Array"=w295:string[])  [unwired: 9 in, 1 out]
        n180 = Build Array (concatenate)("Select the test to run...", w295) -> (w294:string[])
        n181 = property on="Test Name" class="Ring (strict)"("Strings []"=w294) -> ()  [unwired: 2 in, 2 out]
      }
      event "Test Name": Value Change {
        w297 = FALSE ("Visible")
        # "Tell the robot the test name to run"
        n182 = event-data() -> ("NewVal"=w301:u16)  [unwired: 1 in]
        n183 = property on="Test Name" class="Ring (strict)"() -> ("Strings []"=w302:string[])  [unwired: 2 in, 2 out]
        n184 = local write "Progress"(T7 {"Test Progress"=0, "Test Progress Text"=""} ("Progress")) -> ()
        n185 = Index Array(array=w302, index=w301) -> (element=w300:string)
        n186 = call <vilib>:"NT Write String.vi"("String"=w300, "Name"="TestMode/TestName") -> ()  [unwired: 9 in, 1 out]
        n187 = property on="Progress" class="Clust (strict)"("Visible"=TRUE) -> ()  [unwired: 2 in, 2 out]
        n188 = property on="Motor" class="Clust (strict)"("Visible"=w297) -> ()  [unwired: 2 in, 2 out]
        n189 = property on="Test Slider" class="Slide (strict)"("Visible"=w297) -> ()  [unwired: 2 in, 2 out]
        n190 = property on="On/Off" class="Bool (strict)"("Visible"=w297) -> ()  [unwired: 2 in, 2 out]
        n191 = property on="Rev/Fwd" class="Clust (strict)"("Visible"=w297) -> ()  [unwired: 2 in, 2 out]
        n192 = property on="Test Ring" class="Ring (strict)"("Visible"=w297) -> ()  [unwired: 2 in, 2 out]
      }
      event "Listbox": Double Click {
        n193 = event-data() -> ("PlatMods.Shift"=w305:bool, "Row"=w307:i32)  [unwired: 1 in]
        n194 = case shown="True" w305 {
          tunnel: w307 -> [w311 _]
          tunnel: 1 -> [w310 _]
          frame False {
            n195 = property on="Listbox" class="LstBox (strict)"() -> ("Item Symbols"=w309:i32[])  [unwired: 2 in, 2 out]
            n196 = Replace Array Subset(array=w309, new element=w310, index=w311) -> (w308:i32[])
            n197 = property on="Listbox" class="LstBox (strict)"("Item Symbols"=w308) -> ()  [unwired: 2 in, 2 out]
          }
          frame True {
            w312 = 0 ("Top Row")
            n198 = property on="Listbox" class="LstBox (strict)"() -> ("Number of Rows"=w314:u32)  [unwired: 2 in, 2 out]
            n199 = Initialize Array(0, w314) -> (w313:i32[])
            n200 = property on="Listbox" class="LstBox (strict)"("Top Row"=w312, "Value"=w312, "Item Symbols"=w313) -> ()  [unwired: 2 in, 2 out]
          }
        }
      }
      event "Listbox": Key Down {
        n201 = event-data() -> ("VKey"=w318:T14)  [unwired: 1 in]
        n202 = case shown="\"Left\", \"Right\"" w318 {
          selector: w318 -> [w323 _]
          tunnel: eventvkey."Left" ("VKey") -> [w321 _]
          frame "Left", "Right" {
            n203 = Equal?(x=w321, y=w323) -> (x = y?=w322:bool)
            n204 = Select(t=0, s=w322, f=1) -> (s? t:f=w324:i32)
            n205 = property on="Listbox" class="LstBox (strict)"() -> ("Item Symbols"=w327:i32[])  [unwired: 2 in, 2 out]
            n206 = Replace Array Subset(array=w327, new element=w324, index="Listbox") -> (w326:i32[])
            n207 = property on="Listbox" class="LstBox (strict)"("Item Symbols"=w326) -> ()  [unwired: 2 in, 2 out]
          }
          frame Default {
          }
        }
      }
      event "DB Camera Config": Value Change {
        n208 = event-data() -> ("NewVal"=w331:bool)  [unwired: 1 in]
        n209 = case shown="False" w331 {
          tunnel: w330 -> [w340 _]
          tunnel: [w333 w351] -> w329
          tunnel: w328 -> [w332 w351]
          frame False {
            w347 = "Camera"
            w350 = FALSE ("Visible")
            n210 = local read "Camera Settings"() -> (w339:T2)
            n211 = Index Array(array=w340) -> (element=w343:cluster{string[]})  [unwired: 1 in]
            n212 = Unbundle(w339) -> ("Frame Rate"=w338:i32, "Compression"=w337:i32, "Size"=w341:u16)
            n213 = Unbundle(w343) -> (w342:string[])
            n214 = Index Array(array=w342, index=w341) -> (element=w336:string)
            n215 = call-poly <vilib>:"Write Key.vi"("section"=w347, "value"=w336, "key"="Size", "refnum"=w332) -> ("refnum out"=w349:T13)  [unwired: 2 in, 5 out]
            n216 = call-poly <vilib>:"Write Key.vi"("section"=w347, "value"=w338, "key"="FrameRate", "refnum"=w349) -> ("refnum out"=w348:T13)  [unwired: 1 in, 6 out]
            n217 = property on="Camera Settings" class="Clust (strict)"("Visible"=w350) -> ()  [unwired: 2 in, 2 out]
            n218 = local write "DB Camera Config"(w350) -> ()
            n219 = call-poly <vilib>:"Write Key.vi"("section"=w347, "value"=w337, "key"="Compression", "refnum"=w348) -> ("refnum out"=w334:T13)  [unwired: 1 in, 6 out]
            n220 = call <vilib>:"Close Config Data.vi"("refnum"=w334) -> ("file path"=w335:path)  [unwired: 2 in, 8 out]
            n221 = call <vilib>:"Open Config Data.vi"("configuration file path"=w335) -> ("refnum"=w333:T13)  [unwired: 8 in, 2 out]
          }
          frame True {
            n222 = property on="Camera Settings" class="Clust (strict)"("Visible"=TRUE) -> ()  [unwired: 2 in, 2 out]
          }
        }
      }
      event "Camera Settings": Value Change {
        n223 = event-data() -> ("NewVal"=w364:T2)  [unwired: 1 in]
        n224 = Index Array(array=w360) -> (element=w359:cluster{string[]})  [unwired: 1 in]
        n225 = Unbundle(w364) -> ("Frame Rate"=w355:i32, "Compression"=w354:i32, "Size"=w357:u16)
        n226 = Unbundle(w359) -> (w358:string[])
        n227 = Index Array(array=w358, index=w357) -> (element=w356:string)
        n228 = Format Into String(format string="%s   %dfps   %d%%", w356, w355, w354) -> (resulting string=w361:string)  [unwired: 2 in, 1 out]
        n229 = Build Array(w361) -> (w362:string[])
        n230 = property on="DB Camera Config" class="Bool (strict)"("Strings [4]"=w362) -> ()  [unwired: 2 in, 2 out]
      }
      event "Motor.Enable": Value Change {
        n231 = event-data() -> ("NewVal"=w370:bool)  [unwired: 1 in]
        n232 = Unbundle("Motor") -> ("Value"=w369:dbl)  [unwired: 1 out]
        n233 = Select(t=w369, s=w370, f=0.0) -> (s? t:f=w367:dbl)
        n234 = call <vilib>:"NT Write Number.vi"("Numeric"=w367, "Name"=w366) -> ()  [unwired: 9 in, 1 out]
      }
      event "Test Slider": Value Change {
        n235 = event-data() -> ("NewVal"=w373:dbl)  [unwired: 1 in]
        n236 = call <vilib>:"NT Write Number.vi"("Numeric"=w373, "Name"=w374) -> ()  [unwired: 9 in, 1 out]
      }
      event "On/Off": Value Change {
        n237 = event-data() -> ("NewVal"=w378:bool)  [unwired: 1 in]
        n238 = Boolean To (0,1)(Boolean=w378) -> (0, 1=w377:i16)
        n239 = call <vilib>:"NT Write Number.vi"("Numeric"=w377, "Name"=w376) -> ()  [unwired: 9 in, 1 out]
      }
      event "Rev/Fwd": Value Change {
        n240 = event-data() -> ("NewVal.Forward"=w386:bool, "NewVal.Reverse"=w385:bool)  [unwired: 1 in]
        n241 = Boolean To (0,1)(Boolean=w386) -> (0, 1=w382:i16)
        n242 = Boolean To (0,1)(Boolean=w385) -> (0, 1=w384:i16)
        n243 = Negate(x=w384) -> (-x=w383:i16)
        n244 = Add(x=w382, y=w383) -> (x+y=w381:i16)
        n245 = call <vilib>:"NT Write Number.vi"("Numeric"=w381, "Name"=w380) -> ()  [unwired: 9 in, 1 out]
      }
      event "Test Ring": Value Change {
        n246 = event-data() -> ("NewVal"=w390:u16)  [unwired: 1 in]
        n247 = property on="Test Ring" class="Ring (strict)"() -> ("Strings []"=w391:string[])  [unwired: 2 in, 2 out]
        n248 = Index Array(array=w391, index=w390) -> (element=w389:string)
        n249 = call <vilib>:"NT Write String.vi"("String"=w389, "Name"=w388) -> ()  [unwired: 9 in, 1 out]
      }
      event "Rec Mode": Value Change {
        # "Update globals for recording mode and path to read log from.\nClear when logging and let NetworkTables set path for vision to\nuse."
        n250 = event-data() -> ("NewVal"=w401:enum32{"Stop", "Record", "Playback"})  [unwired: 1 in]
        n251 = global write "WPI_DashboardLogging Global.vi" "Logging Filename"(path "") -> ()
        n252 = case shown="\"Stop\", \"Record\"" w401 {
          tunnel: w400 -> [_ w403 w411]
          tunnel: [_ _ w410] -> w397
          tunnel: [_ _ w409] -> _
          tunnel: w395 -> [_ _ w407]
          tunnel: cluster{i32, i32} {-250, 170} -> [_ _ w406]
          tunnel: [_ _ T15 {"Image Size"=TRUE, "Image Type"=TRUE, "Pixel Value"=TRUE, "ROI Information"=TRUE, "Zoom Factor"=FALSE} ("Image Information Shown:All Elements")] -> w393
          tunnel: [_ _ TRUE ("Zoom Factor")] -> w392
          frame Default {
          }
          frame "Stop", "Record" {
            # "Place Window too"
            n253 = invoke class="VI" method="FP.Close"(reference=w403) -> (reference out=w402:refnum<vi>)  [unwired: 2 in, 2 out]
            n254 = invoke class="VI" method="Abort VI"(reference=w402) -> ()  [unwired: 2 in, 3 out]
          }
          frame "Playback" {
            n255 = call "Open Playback Panel.vi"("Offset"=w406, "DB VI Ref"=w407, "Playback in"=w411) -> ("Playback out"=w408:refnum<vi>)  [unwired: 8 in]
            n256 = register-events(w408) -> (reference out=w410:refnum<event-registration>, error out=w409:errorcluster)  [unwired: 2 in]
          }
        }
        n257 = global write "WPI_DashboardLogging Global.vi" "Recording"(w401) -> ()
        n258 = property on="Camera Image" class="ImageControl"("Image Information Shown"=w393, "Image Information Visible"=w392) -> ()  [unwired: 2 in, 2 out]
        n259 = call <vilib>:"WPI_DashboardNT Log FieldName Cache.vi"("Operation"=enum16{"Lookup/Add", "Index", "Clear"}."Clear") -> ()  [unwired: 8 in, 3 out]
      }
      event Panel Close {
        w412 = enum32{"Stop", "Record", "Playback"}."Stop" ("Rec Mode")
        n260 = event-data() -> ()  [unwired: 1 in, 4 out]
        n261 = local write "Rec Mode"(w412) -> ()
        n262 = global write "WPI_DashboardLogging Global.vi" "Recording"(w412) -> ()
      }
      event Panel Close {
        # "Abort playback window and ourself"
        n263 = event-data() -> ()  [unwired: 1 in, 4 out]
        n264 = invoke class="VI" method="FP.Close"(reference=w417) -> (reference out=w416:refnum<vi>)  [unwired: 2 in, 2 out]
        n265 = invoke class="VI" method="Abort VI"(reference=w416) -> (error out=w415:errorcluster)  [unwired: 2 in, 2 out]
        n266 = invoke class="VI" method="Abort VI"(error in=w415) -> ()  [unwired: 2 in, 3 out]
      }
    }
  }
  n267 = property on="On/Off" class="Bool (strict)"("Visible"=w25) -> ()  [unwired: 2 in, 2 out]
  n268 = property on="Motor" class="Clust (strict)"("Visible"=w25) -> ()  [unwired: 2 in, 2 out]
  n269 = property on="Progress" class="Clust (strict)"("Visible"=w25) -> ()  [unwired: 2 in, 2 out]
  n270 = property on="Test Ring" class="Ring (strict)"("Visible"=w25) -> ()  [unwired: 2 in, 2 out]
  n271 = property on="Rev/Fwd" class="Clust (strict)"("Visible"=w25) -> ()  [unwired: 2 in, 2 out]
  n272 = property on="Camera Settings" class="Clust (strict)"("Visible"=w25) -> ()  [unwired: 2 in, 2 out]
  n273 = local write "DB Camera Config"(w25) -> ()
  n274 = global write "WPI_DashboardLogging Global.vi" "Recording"(w8) -> ()
  n275 = local write "Rec Mode"(w8) -> ()
